vi "SaveParams.vi"(9 "NormalType":bool, 10 "Params":string[][](table), 11 "FundParams":string[][](table)) -> (3 "PmuTestParams":T1)   [LabVIEW 2018, in "Functions.lvlib" / "PmuTestFunctions.lvclass"]
uses:
  PmuTestFunctions.lvclass
  Typedefs/PmuTestParams.ctl
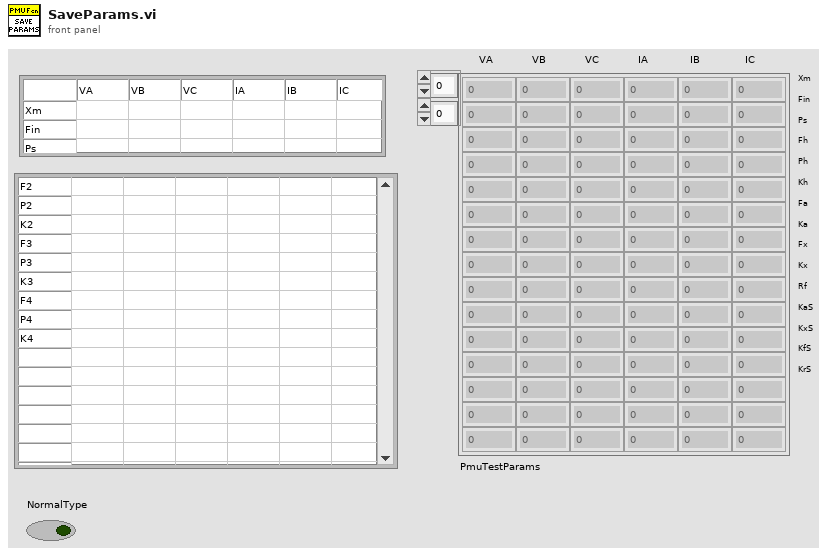
[diagram p1: front panel]
types:
  T1 = typedef "Functions.lvlib/PmuTestFunctions.lvclass/PmuTestParams.ctl" = dbl[][]
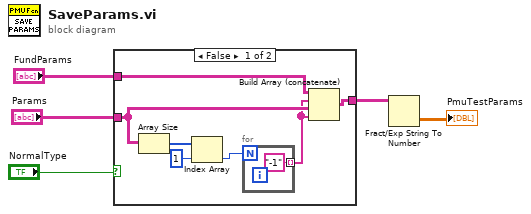
[diagram p0: block diagram]
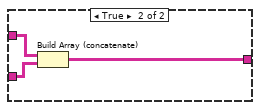
[diagram p2: hidden frame]
diagram:
  n1 = case shown="False" "NormalType" {
    tunnel: "Params" -> [w7 w15]
    tunnel: "FundParams" -> [w9 w16]
    tunnel: [w8 w14] -> w2
    frame False {
      n2 = Array Size(array=w7) -> (size(s)=w12:i32[])
      n3 = Index Array(array=w12, index=1) -> (element=w10:i32)
      n4 = for {
        N: w10 -> [_]
        tunnel: ["-1"] -> w6 mode=indexing
      }
      n5 = Build Array (concatenate)(w9, w6, w7, w6) -> (w8:string[][])
    }
    frame True {
      n6 = Build Array (concatenate)(w16, w15) -> (w14:string[][])
    }
  }
  n7 = Fract/Exp String To Number(string=w2) -> (number=→"PmuTestParams":dbl[][])  [unwired: 3 in, 1 out]
